vi "Generate State Information.vi"(8 "error in (no error)":errorcluster, 11 "JSON RCT":refnum<class "JSON Routing Channel Template.lvclass">) -> (0 "error out":errorcluster, 2 "State Configurations":T1[](array[typedef])=[{"Name"="No Connections", "Description"="State with no connections", "Value"=-1, "Connection List"=[]}], 3 "JSON RCT":refnum<class "JSON Routing Channel Template.lvclass">)   [LabVIEW 2020, in "Routing Templates.lvlib" / "JSON Routing Channel Template.lvclass"]
uses:
  JSON Routing Channel Template.lvclass
  JSON Routing Channel Template.lvclass/JSON Routing Channel Template.ctl
  Shared/Connection.ctl
  Shared/Routing and Faulting Shared.lvlib
  Shared/Routing State.ctl
  Connection Lookups/Abstract Connection Lookup/Abstract Connection Lookup.lvclass
  <vilib>/ErrorRing/Error Ring.xnode
  <vilib>/Utility/error.llb/Error Cluster From Error Code.vi
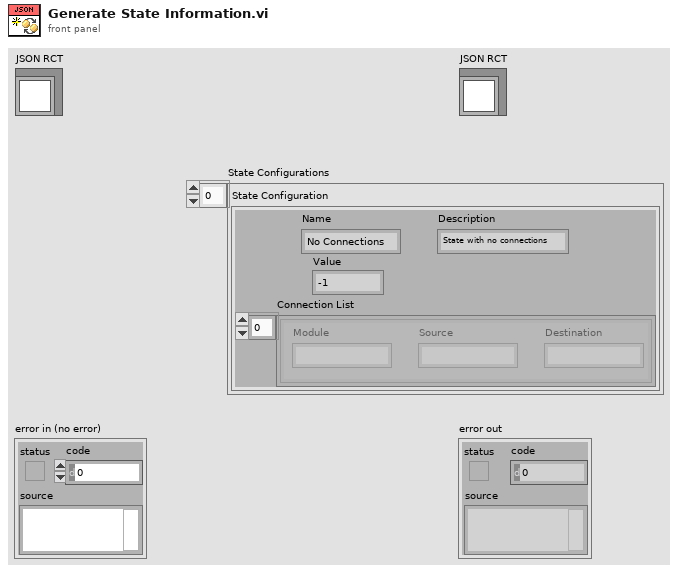
[diagram p1: front panel]
types:
  T1 = typedef "Routing and Faulting Shared.lvlib/Routing State.ctl" = cluster{"Name":string, "Description":string, "Value":i32, "Connection List":T2[]}
  T2 = typedef "Routing and Faulting Shared.lvlib/Connection.ctl" = cluster{"Module":string, "Source":string, "Destination":string}
  T3 = cluster{"Name":string, "Description":string, "Value":i32, "Connection List":cluster{"Channel":string, "Connection Type":string}[]}[]
  T4 = cluster{"Channel":string, "Connection Type":string}[]
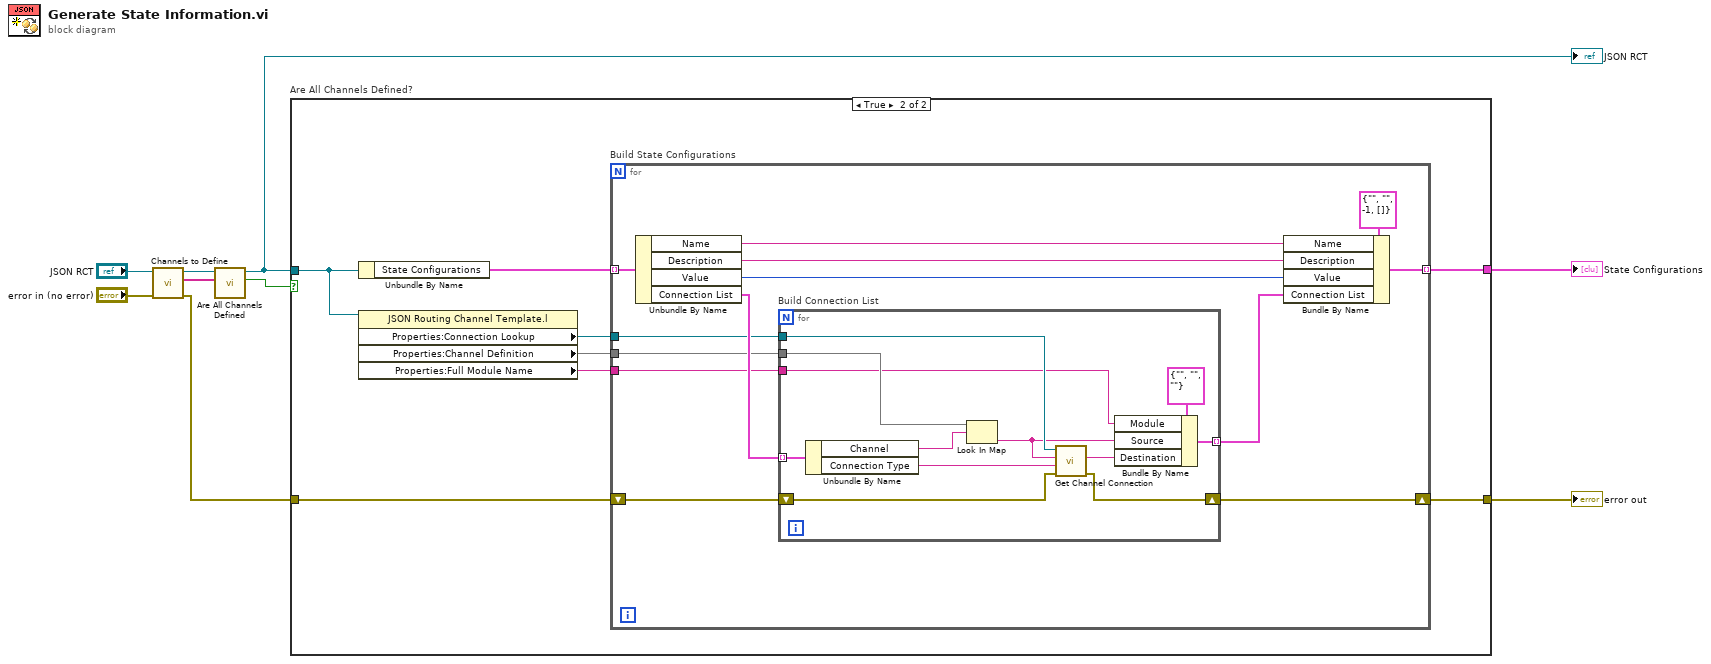
[diagram p0: block diagram]
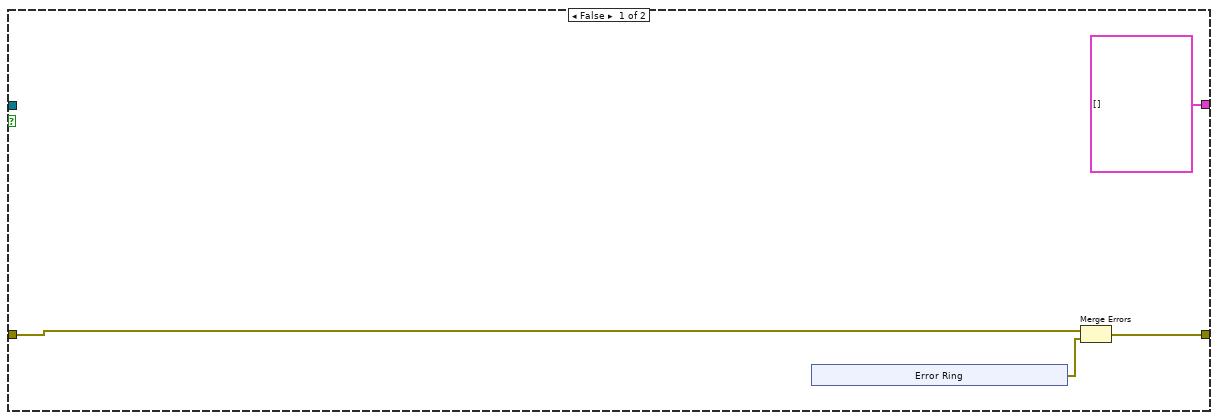
[diagram p2: hidden frame]
diagram:
  n1 = call-dynamic "Channels to Define.vi"("error in (no error)"="error in (no error)", "JSON Routing Channel Template in"="JSON RCT") -> ("error out"=w2:errorcluster, "Channels"=w6:string[], "JSON Routing Channel Template out"=w7:refnum<class "JSON Routing Channel Template.lvclass">)  [unwired: 7 in]
  n2 = call "Are All Channels Defined.vi"("Channels"=w6, "JSON RCT"=w7) -> ("All Defined?"=w1:bool, "JSON RTC"=w3:refnum<class "JSON Routing Channel Template.lvclass">)  [unwired: 8 in]
  "JSON RCT" <- w3
  n3 = case "Are All Channels Defined?" shown="True" w1 {
    tunnel: [T1[] [] w25] -> w9
    tunnel: [w12 w23] -> w8
    tunnel: w3 -> [_ w20]
    tunnel: w2 -> [w11 w19]
    frame False {
      n4 = xnode "Error Ring"() -> ("error out"=w10:errorcluster)
      n5 = Merge Errors(w11, w10) -> (w12:errorcluster)
    }
    frame True {
      n6 = Unbundle By Name(w20) -> ("State Configurations"=w26:T3)
      n7 = property class="JSON Routing Channel Template.l"(reference=w20) -> ("Properties:Connection Lookup"=w24:refnum<class "Abstract Connection Lookup.lvclass">, "Properties:Channel Definition"=w22:map{string, string}, "Properties:Full Module Name"=w21:string)  [unwired: 1 in, 2 out]
      n8 = for "Build State Configurations" {
        tunnel: w26 -> [w38] mode=indexing
        tunnel: [w34] -> w25 mode=indexing
        tunnel: w24 -> [w29]
        shift-right: [w30] -> w23
        shift-left: w19 -> [w31]
        tunnel: w22 -> [w28]
        tunnel: w21 -> [w27]
        n9 = Unbundle By Name(w38) -> ("Name"=w37:string, "Description"=w36:string, "Value"=w35:i32, "Connection List"=w33:T4)
        n10 = for "Build Connection List" {
          tunnel: w33 -> [w49] mode=indexing
          tunnel: [w50] -> w32 mode=indexing
          shift-right: [w46] -> w30
          shift-left: w31 -> [w47]
          tunnel: w29 -> [w44]
          tunnel: w28 -> [w43]
          tunnel: w27 -> [w40]
          n11 = Unbundle By Name(w49) -> ("Channel"=w42:string, "Connection Type"=w48:string)
          n12 = Look In Map(map=w43, key=w42) -> (value=w41:string)  [unwired: 1 in, 1 out]
          n13 = call-dynamic "Get Channel Connection.vi"("error in (no error)"=w47, "Connection Type"=w48, "Channel"=w41, "Abstract Connection Lookup in"=w44) -> ("error out"=w46:errorcluster, "Connected Channel"=w45:string)  [unwired: 5 in, 1 out]
          n14 = Bundle By Name(cluster=T2 {"Module"="", "Source"="", "Destination"=""} ("Connection"), "Module"=w40, "Source"=w41, "Destination"=w45) -> (w50:T2)
        }
        n15 = Bundle By Name(cluster=T1 {"Name"="", "Description"="", "Value"=-1, "Connection List"=[]} ("State Configuration"), "Name"=w37, "Description"=w36, "Value"=w35, "Connection List"=w32) -> (w34:T1)
      }
    }
  }
  "error out" <- w8
  "State Configurations" <- w9
